vi "回调函数.vi"(4 "queue out":refnum<queue>, 6 "控件引用":refnum<k7>, 7 "事件通用数据":cluster{"事件源":i32, "事件类型":u32, "时间标识":u32}) -> ()   [LabVIEW 2011]
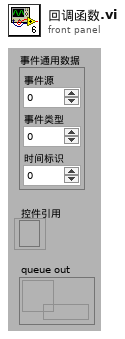
[diagram p1: front panel]
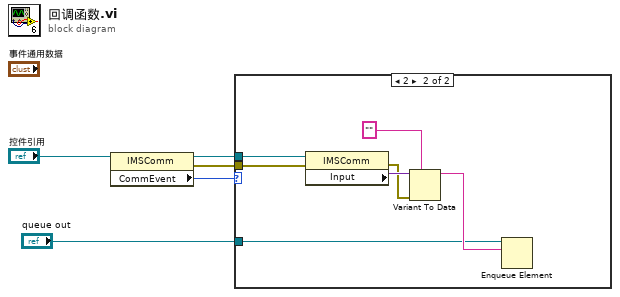
[diagram p0: block diagram]
diagram:
  n1 = property class="IMSComm"(reference="控件引用") -> (reference out=w3:refnum<k7>, error out=w4:errorcluster, "CommEvent"=w5:i16)  [unwired: 1 in]
  n2 = case shown="2" w5 {
    tunnel: w4 -> [_ w12]
    tunnel: w3 -> [_ w11]
    tunnel: "queue out" -> [_ w6]
    frame 0, Default {
    }
    frame 2 {
      n3 = property class="IMSComm"(reference=w11, error in=w12) -> (error out=w8:errorcluster, "Input"=w10:variant)  [unwired: 1 out]
      n4 = Variant To Data(error in=w8, type="", Variant=w10) -> (data=w7:string)  [unwired: 1 out]
      n5 = Enqueue Element(queue=w6, element=w7) -> ()  [unwired: 2 in, 3 out]
    }
  }
